vi "Obtain Test Case.vi"(8 "error in (no error)":errorcluster, 9 "Ignore Inherited Tests?":bool, 10 "Test class and methods":string[](array[string]), 11 "Test Finder":refnum<class "Test Finder.lvclass">) -> (0 "error out":errorcluster, 3 "Test Case":refnum<class "LUnit Test Case.lvclass">)   [LabVIEW 2020, in "Execution UI V2.lvclass"]
doc: "Generates a test case from the given class name and method names. All inputs must refer to methods in one lvclass. If hte class is included itself, all methods in the class will be enabled."
uses:
  Execution UI V2.lvclass
  Framework/Test Case/LUnit Test Case.lvclass
  Framework/Helper Classes/Test Finder/Test Finder.lvclass
  Framework/Test Case/LUnit Test Case.lvclass/LUnit Test Case.ctl
  Execution UI V2.lvclass/Execution UI V2.ctl
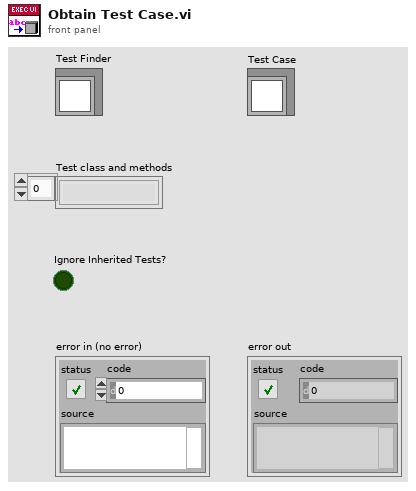
[diagram p1: front panel]
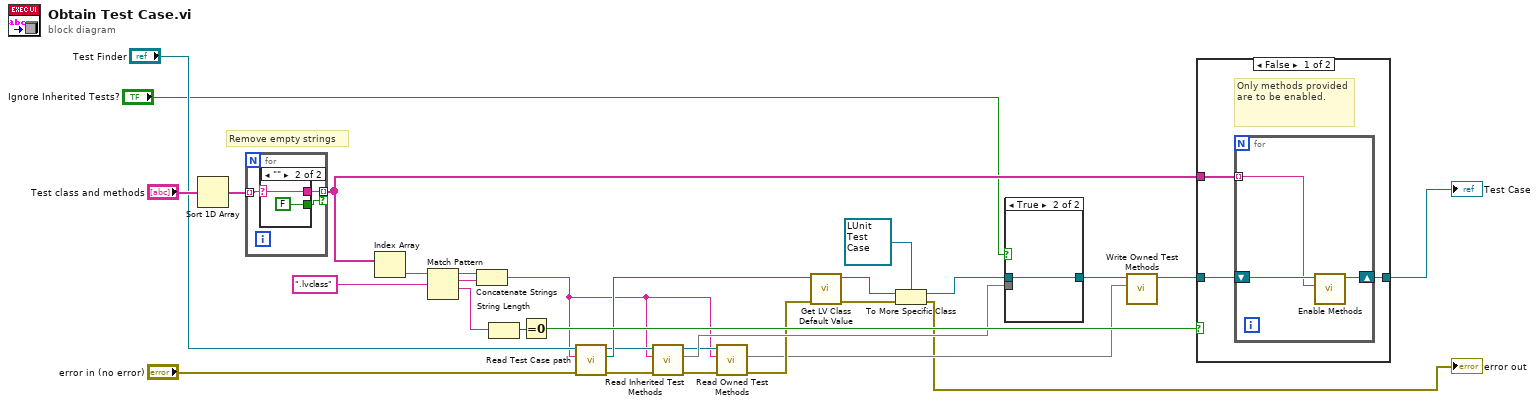
[diagram p0: block diagram]
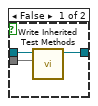
[diagram p2: hidden frame]
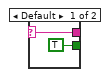
[diagram p4: hidden frame]
diagram:
  # "Remove empty strings"
  n1 = Sort 1D Array(array="Test class and methods") -> (sorted array=w18:string[])
  n2 = for {
    tunnel: w18 -> [w33] mode=indexing
    tunnel: [w32] -> w9 mode=indexing if=w31
    n3 = case shown="\"\"" w33 {
      selector: w33 -> [w35 w37]
      tunnel: [w35 w37] -> w32
      tunnel: [TRUE FALSE] -> w31
      frame Default {
      }
      frame "" {
      }
    }
  }
  n4 = Index Array(array=w9) -> (element=w23:string)  [unwired: 1 in]
  n5 = Match Pattern(string=w23, regular expression=".lvclass") -> (before substring=w22:string, match substring=w21:string, after substring=w25:string)  [unwired: 1 in, 1 out]
  n6 = Concatenate Strings(w22, w21) -> (w3:string)
  n7 = String Length(string=w25) -> (length=w26:i32)
  n8 = Equal To 0?(x=w26) -> (x = 0?=w20:bool)
  n9 = call "Read Test Case path.vi"("error in (no error)"="error in (no error)", "Test Case Name"=w3, "Test Case Finder In"="Test Finder") -> ("error out"=w12:errorcluster, "Class path"=w15:path, "Test Case Finder Out"=w13:refnum<class "Test Finder.lvclass">)  [unwired: 5 in, 1 out]
  n10 = call "Read Inherited Test Methods.vi"("error in (no error)"=w12, "Test Case"=w3, "Test Case Finder In"=w13) -> ("error out"=w11:errorcluster, "Dynamic Test Methods"=w10:map{string, path}, "Test Case Finder Out"=w7:refnum<class "Test Finder.lvclass">)  [unwired: 6 in]
  n11 = call "Read Owned Test Methods.vi"("error in (no error)"=w11, "Test Case"=w3, "Test Case Finder In"=w7) -> ("error out"=w8:errorcluster, "Static Test Methods"=w4:map{string, path})  [unwired: 6 in, 1 out]
  n12 = call <vilib>:"Get LV Class Default Value.vi"("error in (no error)"=w8, "class path"=w15) -> ("error out"=w28:errorcluster, "object"=w27:refnum<class>)  [unwired: 8 in]
  n13 = To More Specific Class(target class=refnum<class "LUnit Test Case.lvclass"> refnum ("Test Case.lvclass"), reference=w27, error in=w28) -> (specific class reference=w14:refnum<class "LUnit Test Case.lvclass">, error out=→"error out":errorcluster)
  n14 = case shown="True" "Ignore Inherited Tests?" {
    tunnel: w14 -> [w40 w41]
    tunnel: w10 -> [w39 _]
    tunnel: [w38 w41] -> w6
    frame False {
      n15 = call "Write Inherited Test Methods.vi"("Inherited Test Methods"=w39, "LUnit Test Case In"=w40) -> ("LUnit Test Case Out"=w38:refnum<class "LUnit Test Case.lvclass">)  [unwired: 9 in]
    }
    frame True {
    }
  }
  n16 = call "Write Owned Test Methods.vi"("Owned Test Methods"=w4, "LUnit Test Case In"=w6) -> ("LUnit Test Case Out"=w5:refnum<class "LUnit Test Case.lvclass">)  [unwired: 9 in]
  n17 = case shown="False" w20 {
    tunnel: [w44 w48] -> w30
    tunnel: w5 -> [w43 w48]
    tunnel: w9 -> [w42 _]
    frame False {
      # "Only methods provided are to be enabled."
      n18 = for {
        tunnel: w42 -> [w46] mode=indexing
        shift-right: [w45] -> w44
        shift-left: w43 -> [w47]
        n19 = call "Enable Methods.vi"("Method"=w46, "LUnit Test Case In"=w47) -> ("LUnit Test Case Out"=w45:refnum<class "LUnit Test Case.lvclass">)  [unwired: 9 in]
      }
    }
    frame True {
      # "The class included in the list -> Do not filter methods"
    }
  }
  "Test Case" <- w30
